vi "Workspace.Select.Dialog.vi"(10 "CD Path":string, 11 "NIVS.System Definition Root":refnum<k24>) -> (1 "Cancelled?":bool, 2 "IP Address":string="Targets/Controller/Custom Devices/Communication Example", 3 "Custom Device Path Out":string="Targets/Controller/Custom Devices/Communication Example")   [LabVIEW 2024, in "Diagnostics Workspace Shared.lvlib"]
uses:
  Diagnostics Workspace Shared.lvlib
  NationalInstruments.VeriStand.SystemStorage
panel:
  in  "Cancel":bool
  in  "Select":bool
  in  "Custom Device Path":string(tree)
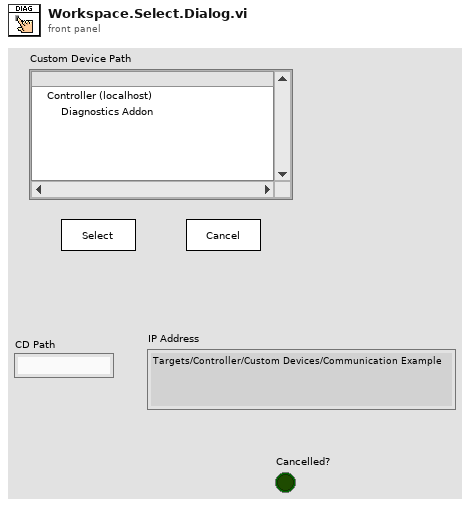
[diagram p1: front panel]
types:
  T1 = enum8{"Enabled", "Disabled", "Disabled and Grayed Out"}
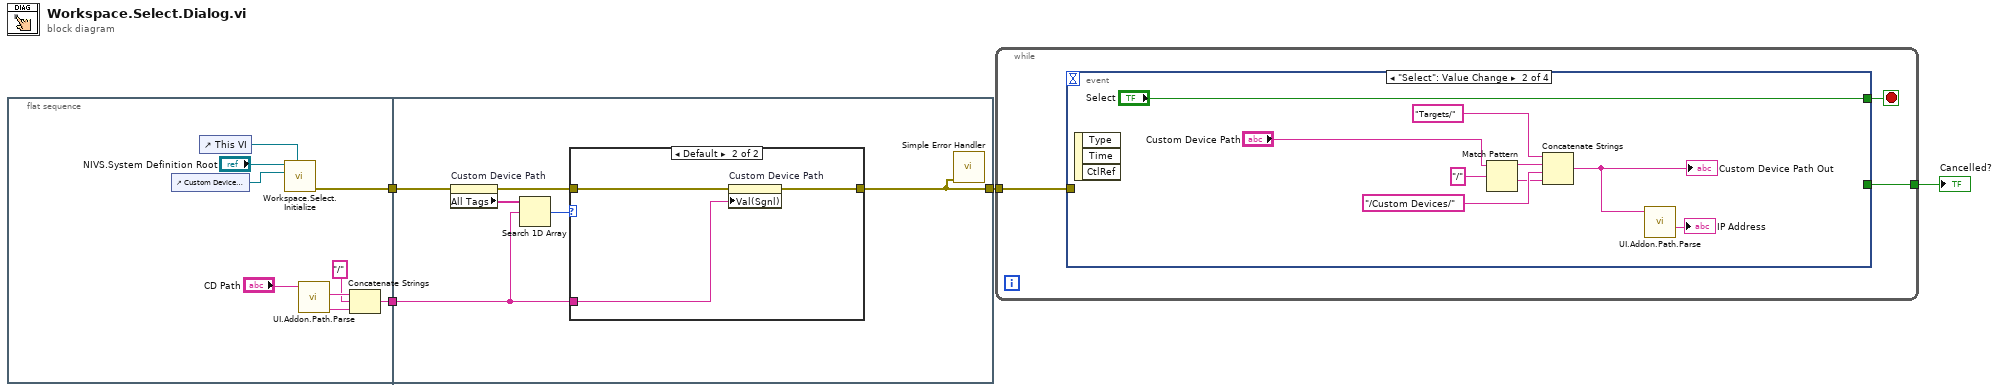
[diagram p0: block diagram]
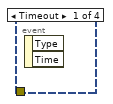
[diagram p2: hidden frame]
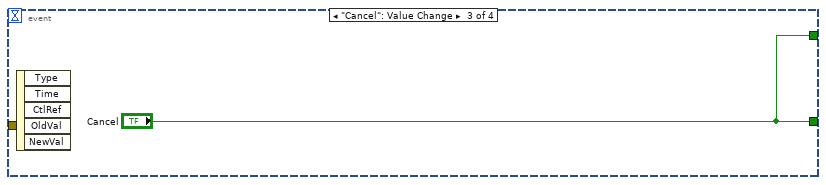
[diagram p3: hidden frame]
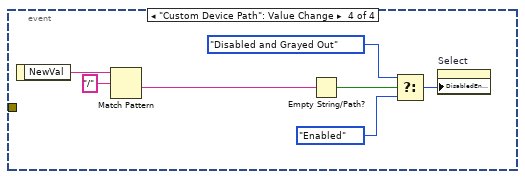
[diagram p4: hidden frame]
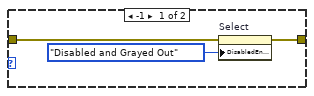
[diagram p5: hidden frame]
diagram:
  n1 = flat-sequence {
    tunnel: [w11] -> w3
    tunnel: [w9] -> w1
    tunnel: [w19] -> w4
    tunnel: w3 -> [w18]
    tunnel: w1 -> [w15]
    frame #0 {
      n2 = control-ref of="Custom Device Path"() -> (w12:refnum<vi>)
      n3 = control-ref of="This VI"() -> (w10:refnum<vi>)
      n4 = call "Workspace.Select.Initialize.vi"("VI reference (current VI)"=w10, "Tree"=w12, "NIVS.System Definition Root"="NIVS.System Definition Root") -> ("error out"=w11:errorcluster)  [unwired: 7 in, 1 out]
      n5 = call "UI.Addon.Path.Parse.vi"("Cached Addon Path"="CD Path") -> ("Addon Name"=w6:string, "Controller and IP Address"=w7:string)  [unwired: 6 in, 3 out]
      n6 = Concatenate Strings(w7, "/" ("regular expression"), w6) -> (w9:string)
    }
    frame #1 {
      n7 = property on="Custom Device Path" class="Tree (strict)"(error in=w18) -> (error out=w17:errorcluster, "All Tags"=w16:string[])  [unwired: 1 in, 1 out]
      n8 = Search 1D Array(1D array=w16, element=w15) -> (index of element=w14:i32)  [unwired: 1 in]
      n9 = case shown="Default" w14 {
        tunnel: [w22 w25] -> w19
        tunnel: w17 -> [w21 w24]
        tunnel: w15 -> [_ w23]
        frame -1 {
          n10 = property on="Select" class="Bool"(error in=w21, "DisabledEnum"=T1."Disabled and Grayed Out" ("Disabled")) -> (error out=w22:errorcluster)  [unwired: 1 in, 1 out]
        }
        frame Default {
          n11 = property on="Custom Device Path" class="Tree (strict)"(error in=w24, "Val(Sgnl)"=w23) -> (error out=w25:errorcluster)  [unwired: 1 in, 1 out]
        }
      }
      n12 = call <vilib>:"Simple Error Handler.vi"("error in (no error)"=w19) -> ()  [unwired: 4 in, 5 out]
    }
  }
  n13 = while {
    tunnel: w4 -> [w28]
    tunnel: [w26] -> w2
    stop <- w27 stop-if-true
    n14 = event shown="[1] \"Select\": Value Change" {
      selector: _ -> [_ _ _ _]
      dyn-events: _ -> [_ _ _ _]
      timeout: _ -> [_ _ _ _]
      tunnel: w28 -> [_ _ _ _]
      tunnel: [_ "Select" "Cancel" _] -> w27
      tunnel: [_ _ "Cancel" _] -> w26
      event Timeout {
        n15 = event-data() -> ()  [unwired: 1 in, 2 out]
      }
      event "Select": Value Change {
        n16 = event-data() -> ()  [unwired: 1 in, 3 out]
        n17 = Match Pattern(string="Custom Device Path", regular expression="/") -> (before substring=w35:string, after substring=w33:string)  [unwired: 1 in, 2 out]
        n18 = Concatenate Strings("Targets/" ("string"), w35, "/Custom Devices/" ("string"), w33) -> (w29:string)
        "Custom Device Path Out" <- w29
        n19 = call "UI.Addon.Path.Parse.vi"("Cached Addon Path"=w29) -> ("IP Address"=→"IP Address":string)  [unwired: 6 in, 4 out]
      }
      event "Cancel": Value Change {
        n20 = event-data() -> ()  [unwired: 1 in, 5 out]
      }
      event "Custom Device Path": Value Change {
        n21 = event-data() -> ("NewVal"=w45:string)  [unwired: 1 in]
        n22 = Match Pattern(string=w45, regular expression="/") -> (after substring=w39:string)  [unwired: 1 in, 3 out]
        n23 = Empty String/Path?(string/path=w39) -> (empty?=w44:bool)
        n24 = Select(t=T1."Disabled and Grayed Out" ("Disabled"), s=w44, f=T1."Enabled" ("Disabled")) -> (s? t:f=w41:T1)
        n25 = property on="Select" class="Bool"("DisabledEnum"=w41) -> ()  [unwired: 2 in, 2 out]
      }
    }
  }
  "Cancelled?" <- w2
